vi "2023_day07_Task1.vi"() -> ()   [LabVIEW 2021]
uses:
  11e8d1f3-b77f-4a8a-b28c-9a22c915bc09.vi
  <userlib>/_OpenG.lib/array/array.llb/Sort 1D Array (I32)__ogtk.vi
  <vilib>/Comparison/Less/Less Functor/Less Functor.lvclass
panel:
  out "Task 1":i32
  in  "Switch":bool caption="Ex. Data  vs.  User Data"
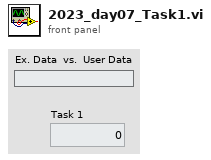
[diagram p1: front panel]
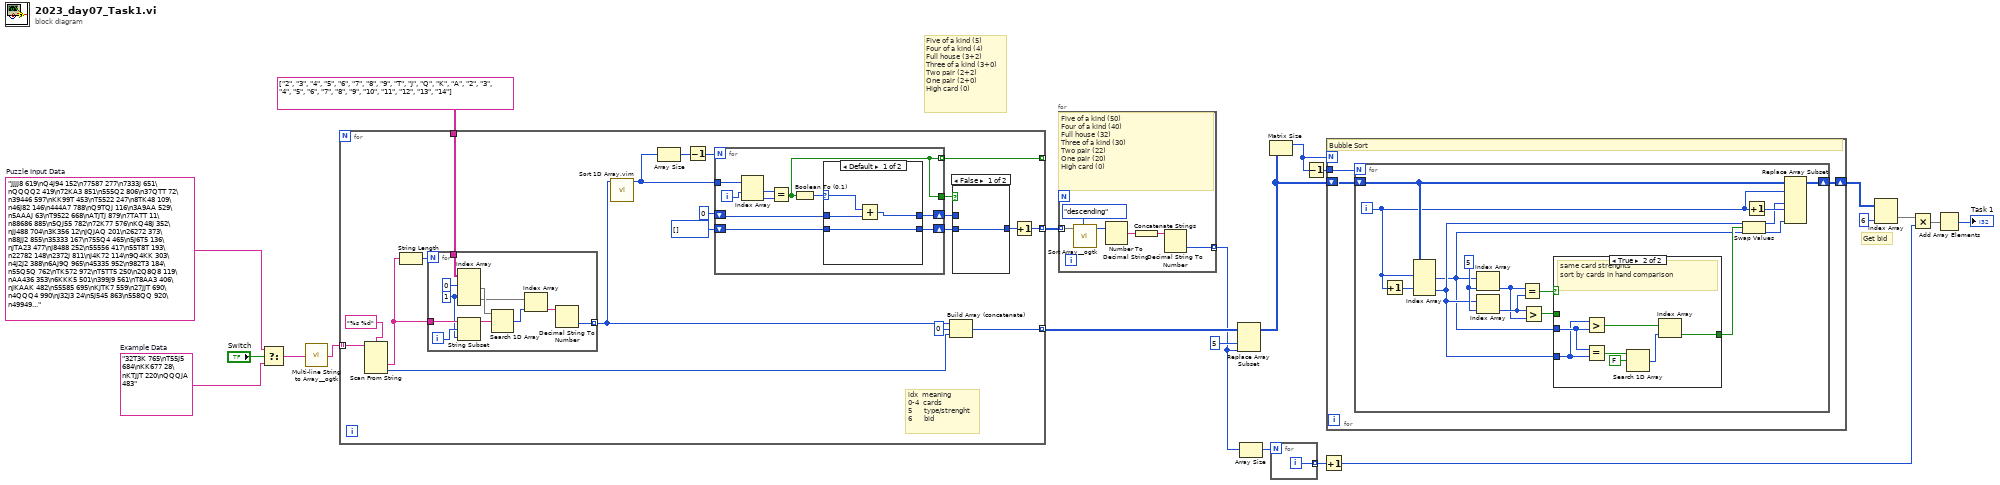
[diagram p0: block diagram]
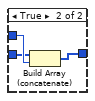
[diagram p3: hidden frame]
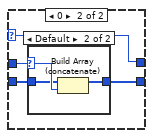
[diagram p4: hidden frame]
diagram:
  w10 = "32T3K 765\nT55J5 684\nKK677 28\nKTJJT 220\nQQQJA 483"  # Example Data
  w20 = "JJJJ8 619\nQ4J94 152\n77587 277\n7333J 651\nQQQQ2 419\n72KA3 851\n555Q2 806\n37QTT 72\n39446 597\nKK99T 453\nT5522 247\n8TK48 109\n46J82 146\n444A7 788\nQ9TQJ 116\n3A9AA 529\n5AAAJ 63\nT9522 668\nATJTJ 879\n7TATT 11\n88686 885\n5QJ55 782\n72K77 576\nKQ48J 352\nJJ488 704\n3K356 12\nJQJAQ 201\n26272 373\n88JJ2 855\n35333 167\n755Q4 465\n5J6T5 136\nJTA23 477\nJ8488 252\n55556 417\n55T8T 193\n22782 148\n2372J 811\nJ4K72 114\n9Q4KK 303\n4J2J2 388\n6AJ9Q 965\n45335 952\n982T3 184\n55Q5Q 762\nTK572 972\nT5TT5 250\n2Q8Q8 119\nAA436 353\n6KKK5 501\n399J9 561\nT8AA3 406\nJKAAK 482\n55585 695\nKJTK7 559\n27JJT 690\n4QQQ4 990\nJ32J3 24\n5J545 863\n558QQ 920\n49949 187\nJQQK9 179\nT29JK 605\n699J6 445\nKK7QJ 284\n647AJ 509\nKK8K3 893\n7KK79 174\nJ8J55 523\n6T3AQ 410\n44349 296\nJJJJJ 158\n99998 570\n5TKQ6 266\n9933T 300\nK665K 724\nQTTTQ 807\n7Q5Q5 375\nQ6666 966\nTQ35K 825\nT5QQ5 18\nKQ794 802\nK42KT 240\nQKKJJ 97\n77647 504\n87J84 443\nKATTK 666\n52J88 889\n66JKJ 977\n6AQ94 84\n36A78 514\nAA67A 286\n74Q34 490\nQQ8QQ 79\n3K555 323\nQ3JKT 338\n2A222 448\n935JJ 798\n43QTJ 226\n5TA7K 162\n553QQ 420\nQKKQ9 204\n9399K 565\n8T66T 638\n4444Q 83\nJ2223 173\n4T454 639\n4K3K4 454\nQ2255 955\n965JJ 658\nA48K3 409\nJJA22 728\n42242 677\nAKT6J 155\n77774 838\n82AAA 894\n22A6K 775\n59377 235\n6K86J 451\n26AT6 671\n8388J 47\nJJ293 449\n39333 500\n62222 456\n5K55Q 36\nKKK77 773\nQQ739 287\n67686 588\n53329 341\nTQTTT 213\n44224 796\nAAAJA 222\n6KK22 92\nAJK2A 627\n5T858 739\nJ6579 462\nT3933 717\n3AQ82 380\nQ564Q 898\n8QQQ7 470\n93T29 317\n64K67 867\nJTTTT 299\n4499J 714\n6QQ76 435\nAJ979 897\n66KTK 594\n2AA84 178\n8858K 533\nKKKKJ 689\n99393 906\n2A777 711\n33Q78 540\n55566 364\n2AA3A 513\n5KJKK 98\nQ79T9 809\nAKKKK 34\n5932K 349\n88858 198\n52222 307\n944T7 126\nT36Q7 472\nT4444 792\nTTKJT 828\n35652 580\nATQ79 94\nATJTA 518\n3JT52 656\n2TT23 438\n9K497 630\nAQ735 569\n95997 175\n27248 874\n3AKJK 693\n94979 709\n2QQT2 137\n4A598 253\n33JQ2 520\n8A747 457\nK222A 720\n89A99 87\nT8TTA 706\nQ489A 322\nJ4TT4 319\nT5JTK 57\nT7T97 280\nA7A7A 471\n9K583 91\n77887 909\n5JJ55 629\nAJ434 901\nJJ7A9 166\nQ99J9 577\n44T4T 688\nT8J8K 759\n5AJ5A 149\n95599 890\n3Q662 781\nJAJ5A 940\nTTJ3J 676\n88976 203\n4AA4Q 985\n95T53 956\nK3333 595\n52555 544\nAK942 684\n2T548 415\nK66J7 407\nKT7T2 103\n97973 14\n43343 708\n55Q53 422\nA835K 616\nTT589 236\n6322K 186\nA4K4A 866\n2K563 861\n5J255 591\nQ9Q98 450\nT7796 305\n9K229 258\n9A27J 993\n5QKQJ 224\nT5J5T 161\n3TA3K 464\n558A8 183\nQ333Q 48\nA5A55 771\n34437 182\n8KKKK 95\nJ5696 291\n66K88 914\n33489 661\nKK2TT 498\n59999 877\n7TTTT 492\n5J52K 531\n398K6 783\n99A9T 49\n667TT 86\nAAKK6 928\n2626J 346\n3J675 37\nT8488 268\nKK222 763\n76666 749\n47457 138\nQTTT6 211\nTTT8T 754\n37754 652\n2QK4K 770\n3A3AA 988\nKJ35A 779\n434AA 962\n44JJ4 519\nK2QQQ 133\nJJ77J 662\n89899 292\nAA9AA 10\n3J3J3 329\n477JJ 841\n39Q33 609\n8A26T 431\nTK63J 641\n57595 880\nKQ7QJ 123\nQJJK5 665\n88AKA 566\n73Q67 265\n7673T 904\nQ7Q2A 937\n9223Q 991\nT45A7 386\n96J6A 220\nQK748 859\nQQAQ8 172\n222K2 100\nQQJ7Q 822\n9AK3A 873\n2766A 647\nK4432 402\nTKTTK 77\n24423 915\nJ5423 853\n32243 463\nQ3QQQ 15\n676T6 368\n54555 378\nAJ7A6 192\n9J3JA 139\n2TT3T 393\nQT33A 503\n56684 120\nQ56Q2 786\nK32AT 943\n384A7 780\n44Q4Q 117\n6AJ54 214\n9J9K9 189\n7TKKT 808\n34J8J 360\nAAATA 755\nJQJTA 705\nT9T94 387\n4J445 718\nQ8Q8Q 6\nT652J 745\nQ9272 372\nT9924 936\n3J352 691\n577T5 827\nQQ344 596\n29TTJ 310\n2332T 752\n66J66 217\n999JJ 261\nQ968T 857\n5233K 165\n3K3KA 489\n33T3J 964\nKT3TT 507\nT88TT 244\n55595 350\n6944J 791\n224AT 887\n3447J 30\nT2K86 169\nQ23Q3 556\nKK88K 602\n4AAA6 534\nATA85 626\n8J3KA 699\nKKQKK 931\n4TTTQ 328\nA3684 923\n62AA2 776\n8464K 121\n846K6 944\n6J69J 610\nKK55J 769\n7TKQ2 358\nTQ4TK 93\nJK4A4 698\n842J8 971\nJJ222 129\n8J32J 233\n278K2 674\n68Q8J 727\nA663T 318\n56A5A 64\n7775Q 180\nK568Q 846\n9K8AA 279\nAJTTK 196\nJA254 151\n5Q2A3 913\nA8788 816\n48729 267\nQKQT4 572\nQ4949 953\n43KK3 125\n83676 2\nJ9959 76\nTJTT3 38\n472T5 948\n5T679 511\nJJ52A 293\n7TT99 649\n47467 176\nJ3J5K 844\n8KJKK 982\nAAJJA 961\n6K633 589\n45Q96 208\n6QQQJ 888\n46464 701\nT33JT 52\n625J9 336\nK84T2 20\n54447 246\nT8AT8 118\n827A6 795\n99967 274\nTT44T 61\nAA2KK 784\nQ2AAT 276\nKA9AA 478\n3QJQK 452\nA97JK 551\nK4774 746\nQKKTT 371\n63834 369\nQQ4QQ 163\n54757 835\n7Q436 919\n3AA33 560\n8Q288 546\n99K99 74\nQJ9QA 67\n48888 404\n4KQA3 850\n36872 930\n359T4 426\nT6578 315\n626T6 772\nK79A9 599\n4A9JA 653\n366J6 45\n2T8J7 628\nTTTT3 967\nA426J 202\nQA6T2 760\n7775A 73\n488K7 16\nKTTTT 644\n84JA9 484\n57775 232\nKTQ8T 7\n8JK88 681\n5A5J8 733\n66A66 228\nK28A4 736\n59647 682\n4Q6A5 663\n62226 578\n5T489 26\n6J65T 548\n24725 9\nK35TJ 314\n26A68 455\nJJTTT 907\nAJ285 899\nJQJQJ 927\nQQTJQ 554\nAT235 141\nTJK9J 35\n9666Q 499\n66A76 999\n86K94 947\n495AT 632\nTK385 403\n993KK 530\n38366 625\n4J744 881\nAA777 694\n84994 248\n46Q2A 39\nTT6TJ 751\nA55AA 741\n2Q545 946\nQT238 959\n22A3A 845\n6T9T7 710\nKKJQK 856\n888A8 722\n3899J 239\n969A9 365\nA88A8 62\nA77J7 945\nQ6222 288\n2QQ62 761\nK22TQ 270\n2JJJJ 421\nKTTKJ 678\nJ32A7 787\n58688 8\n55499 814\nKK7KK 425\n9Q97K 82\n53353 804\n5KQJT 590\n67677 963\nK2A9K 747\nA424A 926\nAJ3T3 891\n75A29 132\n5994T 502\nJ8J5K 399\n44JQQ 437\n6AKQ9 670\nJA376 905\nKAKQA 110\n464JA 908\n88228 719\n37773 558\n555K5 27\nKTT38 902\n7J77J 821\nT888T 13\nJ9K4T 497\n7KJK5 738\n7AKQ2 969\nTQQQ5 785\n5TAT2 849\nJT5A5 143\nQAAAQ 496\nQQKKK 231\nT77K7 488\n77TTQ 461\nTAQ69 535\n43T47 933\n8K3KJ 212\n768QQ 573\nA75A5 643\n88JT4 130\nJ2QQ2 444\nKT788 515\n22922 75\n73TJ5 379\n75555 25\n27666 408\nJ4J3T 41\n94Q57 525\nA85A5 273\n66386 526\nJ98KK 618\nA6A64 234\n2KK2K 147\n3KKKK 636\n88JJ8 495\nT5T55 58\nQ959J 734\n9J292 508\n686J8 376\nA5862 309\nJ9T3T 875\n9Q99Q 22\nT773Q 970\nQ3QT6 424\n4455A 466\n77443 469\n49999 405\nQ65AA 655\nTA576 840\nA9999 96\nAA9J9 256\n5999K 941\n28338 423\n797KT 581\n5K55K 819\n7A3KK 613\n7Q77K 434\nKK686 102\n76755 257\nQ4429 185\n922K2 712\nAA4AA 842\nA2AJA 326\n78A3T 40\nT2Q2T 483\n47A7A 249\n54558 703\n6972Q 522\nAJ689 586\nQ3Q5J 669\n5KK65 262\n2A2AA 847\nA62Q7 737\n2KT2K 645\n4K4TJ 929\nAK993 794\n48576 839\nT4683 604\nQ3556 686\n67Q2K 871\nAA665 370\nQ66Q9 925\nJ77Q7 660\nTJAA7 374\nTT6TA 574\nAJJ4A 414\n3TK28 337\n95AKT 864\n777J9 541\n67979 171\n8888J 829\n5QJQ5 345\n884J4 225\nJQK6T 106\n6K6KJ 367\n333A6 89\n59939 506\n4J525 642\n6A765 624\nA282J 852\n2QJQQ 107\nK8822 70\n67KQA 316\n7J8TQ 111\n5555J 837\n42TQ7 112\nJ2J55 886\n2Q9QJ 942\nATATT 778\n7J676 304\n5K8T7 269\n9KJA2 275\n36TJ3 324\nQJ954 976\n58353 960\n59436 42\nAA444 188\n3A333 834\nJK695 973\n39383 394\nA5566 17\n55533 975\n49448 742\nA8KJK 486\nQQQJ9 524\n73T5Q 65\n8T265 441\n44774 206\n8J329 633\n5555Q 823\n76962 195\n2QQTT 648\nKAQ4Q 882\n6K9A3 312\n62JT8 860\nAKAA5 381\n8888K 216\n66622 4\n76JTJ 884\nKKK2K 343\n2A345 685\nJ922A 440\n2AAAA 487\nK49K5 391\n74QJ2 984\n4777Q 750\n76676 553\n5A829 995\n32K22 584\nJ89Q5 181\n66663 646\nJ4857 335\n66462 623\n36A63 593\nT2Q72 620\n44244 330\nQJ4A7 512\n8J8T8 227\n7ATA7 290\n3A993 325\nQQ2Q2 229\nKKQ5Q 134\nKA658 389\nQQ94Q 467\n5636J 592\n49494 59\n27272 460\nT8T98 536\nT2TTJ 215\nTJQ4Q 68\n5J5JJ 321\n48A79 910\n8465J 954\nK734A 71\n9QJ33 101\nAQAJQ 177\n777J7 401\nK9TTT 1\n8A394 532\n7TTJT 748\nAQT7J 355\nJ547T 735\n8882K 398\n33773 916\nJ7477 294\n5QQQ5 935\n9K9T9 50\n45554 606\nJ44JA 427\n6A494 731\nKQK5T 521\n77447 331\n43J33 543\n8592Q 468\nQ62TJ 430\n99AA9 687\nJ26J6 283\nJ7697 587\n44J44 716\n7K7K7 90\n9KJ49 723\n72724 475\nAA77J 831\n33363 621\nQ3QJQ 306\n66QQQ 744\n9AT23 207\n22733 713\nTA67T 883\n4447K 892\n9JA99 598\n45646 69\n58225 537\nTJTT9 797\nJQJQQ 978\n66T6A 219\nTT6TT 124\nJ484Q 344\nTQ32A 836\n6J6J6 29\n97J9J 979\n6J266 622\nAJ96T 218\n72KKK 298\n2A7A2 243\nTJJ7T 758\n8K682 974\n25QKA 411\nQQQ24 862\n56667 245\n56QQQ 43\n477J4 481\nQ7A5J 555\n45T54 545\nTAQQQ 989\n7AAAA 766\n6Q852 951\n84Q39 458\nJKJ42 730\nAT376 313\n2J427 108\n9TQJ6 429\n444AJ 150\n7TQJT 479\nQQJQQ 127\n2K534 547\nA888Q 272\nJAA65 66\n88585 600\nQ92Q9 528\n7TTA7 725\n3JQT8 160\n444A3 800\nJ5558 878\nJQ5K6 608\n827Q3 122\nJ9999 607\nKJQ69 140\nK368J 99\n5T777 721\nK6665 582\n2666A 683\n6668J 817\n79779 221\nJQ9Q5 474\nJ9996 692\n66J76 396\n53577 732\nJATAA 803\n3KJK6 447\n3K37K 439\nTQQT3 1000\n62A64 416\n78295 571\n33334 726\nJ7999 896\n98988 493\n5AQ5J 153\n4QJ44 320\n4JQQQ 168\n55252 385\n33388 615\n29292 679\n2QAKK 327\n48848 702\n4J3T8 476\nQT332 869\n35899 53\n29A9A 308\n77722 777\n685T5 824\n2242J 238\n66QKJ 131\n6K38Q 397\n5K798 400\nA9JK6 793\n255A2 51\n33TTT 557\n6Q6Q6 311\nQ4687 957\nKK67K 820\nT56A3 432\n75A8J 200\n696J6 78\n94954 382\n2Q89J 356\n35A3A 56\n9J977 575\nA65K2 550\nJ6367 32\n27222 194\nKAAKA 348\nAAAA3 395\nTJ7T7 715\nT3Q92 433\nAQ99Q 843\n79957 263\n9899K 986\n64Q26 801\n34A4Q 922\nJ3838 567\nQQQ5Q 667\nJT732 347\nA8QAT 872\n43T7K 413\n4Q445 362\n34T44 491\nA33A7 932\n22T47 340\n25224 281\nK97Q2 485\n77577 949\n466J6 637\n88868 868\n22822 996\n3AAA4 302\n86J8J 997\nQ24Q2 983\n4224T 357\nT9254 826\nQ2777 980\nK5KKA 28\nK8K88 654\n89432 494\n333J3 538\n79T46 428\n25252 255\nTT8T9 998\n425AA 157\n29TAQ 145\n877K7 60\n558Q3 631\n62665 542\nQ5948 442\n683JQ 197\n49483 697\n3K35K 938\n8TT47 601\n44JAT 568\nT29Q4 33\nAKJ9K 264\n7AAA4 549\nT47A6 241\n27A33 3\n3AA3K 260\n6AK9K 516\n9AJ85 113\nK4454 767\nQ63JJ 764\n4AJK2 958\n66266 278\n74869 994\n8KTK8 768\n73A63 19\nA7285 813\nTA9J4 657\nJTQKT 209\nJ7A55 88\nJAA9A 480\n77282 950\n98J88 359\n7K2K2 753\n44494 700\nK9J6T 918\nKJ74J 282\nQKQK4 640\nT6669 743\nA3QAQ 31\n74AAJ 611\n595J9 757\n5JA59 392\n78878 334\nT4TTT 799\n77678 21\n33KKK 832\n7787J 740\nKAKKA 170\n7KQ3Q 870\nKK9K3 858\n63JJ4 351\nT65J9 199\n37895 412\n9J9A8 833\nK3KJ5 765\n785T2 259\nQ3Q38 564\nJJQJA 446\nQ7JK3 527\nQKK86 634\n4653K 812\n3JK78 815\nJ2255 242\n95A52 789\n93539 254\n5K6Q4 205\n444KK 142\n57K75 191\n3T887 154\nJA685 612\nTA9J8 104\n36847 517\nKJQQK 583\n22J2A 865\n66343 774\n44884 128\n779Q9 934\nT3476 790\n4A446 510\nA8AAA 384\n666AJ 390\n64347 921\nQJ8KA 418\nJJQ6T 563\nJ4236 23\nAJJ37 339\n44448 271\nQ6K96 297\n57J55 115\nTTK8K 729\n666AA 377\n24662 251\n4TAAA 135\n83353 659\n2J429 354\n9K9K9 756\nAQQQQ 459\n45445 301\nA775J 912\n38333 237\nT3T88 680\n9Q2Q3 190\n268K3 164\n868Q7 987\n66466 44\nQJJKQ 818\nT48KQ 854\n526J6 363\n69666 295\n55KAA 895\nK75Q4 144\nTKKKA 332\n98699 650\n78828 848\nKT45K 617\n275TA 992\nJ38QA 635\nTKA3K 579\n4Q4Q5 672\n7377T 614\nKT5J7 675\nQA8TJ 903\n2Q66Q 539\n44J46 917\n4K539 968\n3654Q 55\nA33J7 505\n23959 924\nT25JK 664\n33Q88 911\nQ6677 333\n9669K 289\n9782A 81\n66699 876\n6ATAK 552\n87772 223\n5T555 366\n9KK9K 900\n55666 673\n77KKT 105\n55358 156\nAA4AJ 342\n22TJ2 436\n8A448 361\n4KKK4 80\n84J7Q 805\nATQTJ 473\nK92JQ 707\n222J2 981\nKQ7J7 603\n55JJA 46\nQKJAA 696\n842K5 562\nK58K8 5\nT9T5T 939\nTT956 230\n53555 810\nJK8K8 585\nJ795A 85\n4T8T8 54\nQKK77 830\nKKKJJ 210\n9T9J9 383\n6Q464 285\n73257 159"  # Puzzle Input Data
  # "Get bid"
  # "Five of a kind (5)\nFour of a kind (4)\nFull house (3+2)\nThree of a kind (3+0)\nTwo pair (2+2)\nOne pair (2+0)\nHigh card (0)"
  n1 = Select(t=w20, s="Switch", f=w10) -> (s? t:f=w19:string)
  n2 = call <userlib>:"Multi-line String to Array__ogtk.vi"("string"=w19) -> ("lines"=w18:string[])
  n3 = for {
    tunnel: w18 -> [w41] mode=indexing
    tunnel: string[][] [["2", "3", "4", "5", "6", "7", "8", "9", "T", "J", "Q", "K", "A"], ["2", "3", "4", "5", "6", "7", "8", "9", "10", "11", "12", "13", "14"]] -> [w39]
    tunnel: [w36] -> w16 mode=indexing
    tunnel: [w27] -> _ mode=indexing
    tunnel: [w22] -> w15 mode=indexing
    # "idx  meaning\n0-4  cards\n5      type/strenght\n6      bid"
    n4 = Scan From String(format string="%s %d", input string=w41) -> (output 1=w37:string, output 2=w35:i32)  [unwired: 4 in, 3 out]
    n5 = String Length(string=w37) -> (length=w38:i32)
    n6 = for {
      N: w38 -> [_]
      tunnel: w37 -> [w75]
      tunnel: w39 -> [w78]
      tunnel: [w71] -> w33 mode=indexing
      i -> [w69]
      w68 = 1 ("index (row)")
      n7 = Index Array(array=w78, index (row) #1=0 ("index (row)"), index (row) #2=w68) -> (element #1=w76:string[], element #2=w74:string[])  [unwired: 2 in]
      n8 = String Subset(string=w75, offset (0)=w69, length (rest)=w68) -> (substring=w70:string)
      n9 = Search 1D Array(1D array=w76, element=w70) -> (index of element=w73:i32)  [unwired: 1 in]
      n10 = Index Array(array=w74, index=w73) -> (element=w72:string)
      n11 = Decimal String To Number(string=w72) -> (number=w71:i32)  [unwired: 2 in, 1 out]
    }
    n12 = call "Sort 1D Array.vim"("unsorted array"=w33) -> ("sorted array"=w30:i32[])  [unwired: 10 in]
    n13 = Array Size(array=w30) -> (size(s)=w32:i32)
    n14 = Decrement(x=w32) -> (x-1=w31:i32)
    n15 = for {
      N: w31 -> [_]
      tunnel: w30 -> [w55]
      shift-right: [w50] -> w25
      shift-left: i16 0 -> [w49]
      shift-right: [w48] -> w24
      shift-left: i32[] [] -> [w47]
      tunnel: [w46] -> w27 mode=indexing
      tunnel: [w46] -> w26
      i -> [w54]
      n16 = Index Array(array=w55, index #1=w54) -> (element #1=w52:i32, element #2=w53:i32)  [unwired: 1 in]
      n17 = Equal?(x=w52, y=w53) -> (x = y?=w46:bool)
      n18 = Boolean To (0,1)(Boolean=w46) -> (0, 1=w51:i16)
      n19 = case shown="Default" w51 {
        selector: w51 -> [w58 w63]
        tunnel: [w57 w63] -> w50
        tunnel: w49 -> [w59 w62]
        tunnel: [w56 w61] -> w48
        tunnel: w47 -> [w56 w60]
        frame Default {
          n20 = Add(x=w58, y=w59) -> (x+y=w57:i16)
        }
        frame 0 {
          n21 = case shown="Default" w62 {
            selector: w62 -> [_ w67]
            tunnel: [w64 w66] -> w61
            tunnel: w60 -> [w64 w65]
            frame 0 {
            }
            frame Default {
              n22 = Build Array (concatenate)(w65, w67) -> (w66:i32[])
            }
          }
        }
      }
    }
    n23 = Build Array (concatenate)(w33, 0 ("element"), w35) -> (w36:i32[])
    n24 = case shown="False" w26 {
      tunnel: w25 -> [_ w45]
      tunnel: w24 -> [w42 w44]
      tunnel: [w42 w43] -> w23
      frame False {
      }
      frame True {
        n25 = Build Array (concatenate)(w44, w45) -> (w43:i32[])
      }
    }
    n26 = Increment(x=w23) -> (x+1=w22:i32[])
  }
  n27 = for {
    tunnel: w15 -> [w80] mode=indexing
    tunnel: [w79] -> w7 mode=indexing
    # "Five of a kind (50)\nFour of a kind (40)\nFull house (32)\nThree of a kind (30)\nTwo pair (22)\nOne pair (20)\nHigh card (0)"
    n28 = call-poly <userlib>:"Sort Array__ogtk.vi"("Order"=enum16{"ascending", "descending"}."descending", "Array in"=w80) -> ("Sorted Array out"=w84:i32[])  [unwired: 8 in, 1 out]
    n29 = Number To Decimal String(number=w84) -> (decimal integer string=w83:string[])  [unwired: 1 in]
    n30 = Concatenate Strings(w83) -> (w82:string)
    n31 = Decimal String To Number(string=w82) -> (number=w79:i32)  [unwired: 2 in, 1 out]
  }
  n32 = Replace Array Subset(array=w16, new element=w7, index (col)=5 ("disabled index (col)")) -> (w11:i32[][])  [unwired: 1 in]
  n33 = Array Size(array=w7) -> (size(s)=w6:i32)
  n34 = Matrix Size(0:w11) -> (1:w12:i32)  [unwired: 1 out]
  n35 = for {
    N: w6 -> [_]
    tunnel: [w85] -> w5 mode=indexing
    i -> [w85]
  }
  n36 = Decrement(x=w12) -> (x-1=w13:i32)
  n37 = Increment(x=w5) -> (x+1=w3:i32[])
  n38 = for {
    N: w12 -> [_]
    shift-right: [w88] -> w9
    shift-left: w11 -> [w86]
    tunnel: w13 -> [w87]
    # "Bubble Sort"
    n39 = for {
      N: w87 -> [_]
      shift-right: [w102] -> w88
      shift-left: w86 -> [w103]
      i -> [w95]
      w100 = 5 ("disabled index (col)")
      n40 = Increment(x=w95) -> (x+1=w101:i32)
      n41 = Index Array(array=w103, index (row) #1=w95, index (row) #2=w101) -> (element #1=w89:i32[], element #2=w90:i32[])  [unwired: 2 in]
      n42 = Index Array(array=w89, index=w100) -> (element=w97:i32)
      n43 = Index Array(array=w90, index=w100) -> (element=w98:i32)
      n44 = Equal?(x=w97, y=w98) -> (x = y?=w99:bool)
      n45 = Greater?(x=w98, y=w97) -> (0:w94:bool)
      n46 = case shown="True" w99 {
        tunnel: w90 -> [_ w106]
        tunnel: w89 -> [_ w107]
        tunnel: w94 -> [w104 _]
        tunnel: [w104 w105] -> w91
        frame False {
          # "sort by card strenght"
        }
        frame True {
          # "same card strenghts\nsort by cards in hand comparison"
          n47 = Greater?(x=w106, y=w107) -> (0:w111:bool[])
          n48 = Equal?(x=w107, y=w106) -> (x = y?=w109:bool[])
          n49 = Search 1D Array(1D array=w109, element=FALSE) -> (index of element=w110:i32)  [unwired: 1 in]
          n50 = Index Array(array=w111, index=w110) -> (element=w105:bool)
        }
      }
      n51 = Swap Values(12:w90, 13:w91, 14:w89) -> (1:w92:i32[], 3:w93:i32[])
      n52 = Increment(x=w95) -> (x+1=w96:i32)
      n53 = Replace Array Subset(array=w103, new element #1=w92, index (row) #1=w95, new element #2=w93, index (row) #2=w96) -> (w102:i32[][])  [unwired: 2 in]
    }
  }
  n54 = Index Array(array=w9, index (col)=6 ("disabled index (col)")) -> (element=w4:i32[])  [unwired: 1 in]
  n55 = Multiply(x=w4, y=w3) -> (x*y=w2:i32[])
  n56 = Add Array Elements(numeric array=w2) -> (sum=→"Task 1":i32)
